vi "ArrDevMeasActionback.vi"(7 "DevId":i32, 8 "error in (no error)":errorcluster caption="entrée d'erreur (pas d'erreur)", 9 "CurvePointIndex":i32, 10 "AllPointIndex":i32, 11 "Device In":refnum<class "SymphonyCCD.lvclass"> caption="DNL_LabVIEW Object in") -> (0 "error out":errorcluster caption="sortie d'erreur", 1 "ArrDevDat":T1[](array[typedef]), 2 "MeasDatOut":dbl[][](array[numeric]), 3 "Device Out":refnum<class "SymphonyCCD.lvclass"> caption="DNL_LabVIEW Object out")   [LabVIEW 2019, in "SymphonyCCD.lvclass"]
uses:
  SymphonyCCD.lvclass
  C:/Programmes Labview/LabScanV1A/DevicesClass/BaseDevice/BaseDevice.lvclass
  Experiment Class/ArrDevData.ctl
  SymphonyCCD.lvclass/SymphonyCCD.ctl
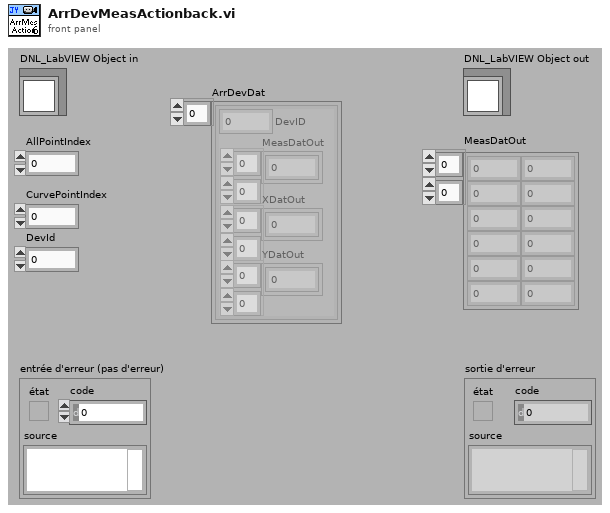
[diagram p1: front panel]
types:
  T1 = typedef "ArrDevData.ctl" = cluster{"MeasDatOut":dbl[][], "XDatOut":dbl[][], "YDatOut":dbl[][], "DevID":i32}
  T2 = cluster{"Message":string, "Data":variant, "Code":i32}
  T3 = typedef "SymphonyCCD.lvclass/SymphonyCCD_Func.ctl" = enum16{"AcqImageSim (Counts)", "AcqImage (Counts)"}
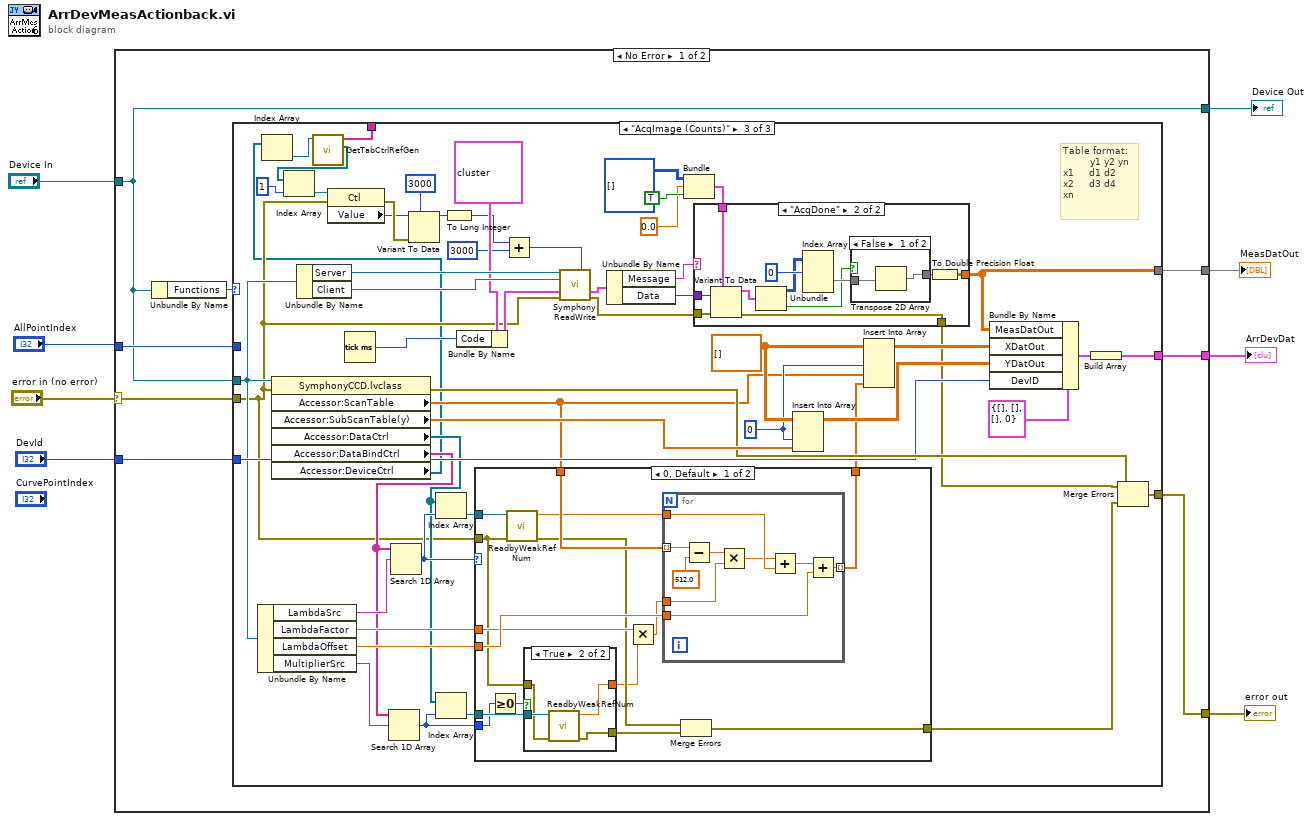
[diagram p0: block diagram]
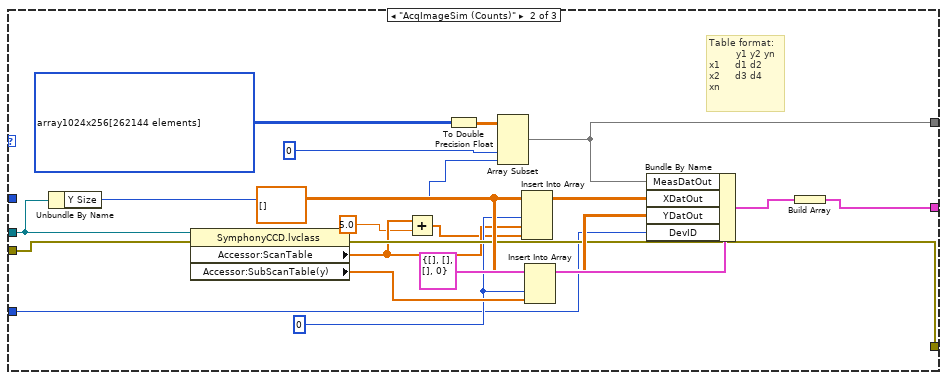
[diagram p3: hidden frame]
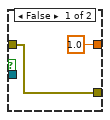
[diagram p4: hidden frame]
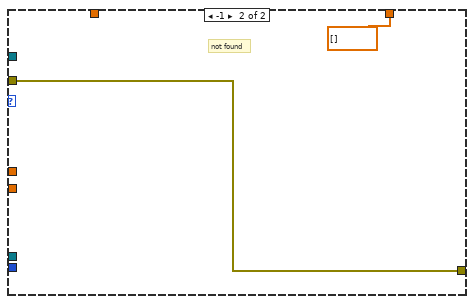
[diagram p5: hidden frame]
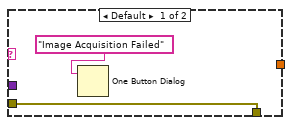
[diagram p6: hidden frame]
diagram:
  n1 = case shown="No Error" "error in (no error)" {
    selector: "error in (no error)" -> [w11 w141]
    tunnel: [w10 w141] -> w8
    tunnel: [w13 w140] -> w6
    tunnel: "Device In" -> [w13 w140]
    tunnel: [w14 _] -> w7
    tunnel: "AllPointIndex" -> [w15 _]
    tunnel: [w12 _] -> w2
    tunnel: "DevId" -> [w9 _]
    frame No Error {
      n2 = Unbundle By Name(w13) -> ("Functions"=w16:T3)
      n3 = case shown="\"AcqImage (Counts)\"" w16 {
        tunnel: w15 -> [_ _ _]
        tunnel: [_ w23 w72] -> w14
        tunnel: w13 -> [_ w26 w64]
        tunnel: [_ w30 w85] -> w12
        tunnel: w11 -> [w17 w29 w48]
        tunnel: [w17 w28 w71] -> w10
        tunnel: w9 -> [_ w21 w82]
        tunnel: [_ _ w39] -> _
        frame Default {
        }
        frame "AcqImageSim (Counts)" {
          w27 = 0 ("indice désactivé (col)")
          w31 = dbl[][] [] ("tableau")
          # "Table format: \n         y1 y2 yn\nx1     d1 d2\nx2     d3 d4\nxn"
          n4 = Unbundle By Name(w26) -> ("Y Size"=w22:i32)
          n5 = property class="SymphonyCCD.lvclass"(reference=w26, error in=w29) -> (error out=w28:errorcluster, "Accessor:ScanTable"=w20:dbl[], "Accessor:SubScanTable(y)"=w32:dbl[])  [unwired: 1 out]
          n6 = Add(x=w20, y=5.0) -> (x+y=w18:dbl[])
          n7 = To Double Precision Float(number=i32[][] array1024x256[262144 elements]) -> (double precision float=w25:dbl[][])
          n8 = Array Subset(array=w25, index (col)=0 ("indice"), length (col)=w22) -> (w23:dbl[][])  [unwired: 2 in]
          n9 = Insert Into Array(array=w31, index (col)=w27, new element #1=w20, new element #2=w18) -> (w34:dbl[][])  [unwired: 1 in]
          n10 = Insert Into Array(array=w31, index (col)=w27, new element=w32) -> (w33:dbl[][])  [unwired: 1 in]
          n11 = Bundle By Name(cluster=T1 {"MeasDatOut"=[], "XDatOut"=[], "YDatOut"=[], "DevID"=0} ("cluster de sortie"), "MeasDatOut"=w23, "XDatOut"=w34, "YDatOut"=w33, "DevID"=w21) -> (w35:T1)
          n12 = Build Array(w35) -> (w30:T1[])
        }
        frame "AcqImage (Counts)" {
          w83 = 0 ("indice désactivé (col)")
          w86 = dbl[][] [] ("tableau")
          # "Table format: \n         y1 y2 yn\nx1     d1 d2\nx2     d3 d4\nxn"
          n13 = Unbundle By Name(w64) -> ("LambdaSrc"=w61:string, "LambdaFactor"=w63:dbl, "LambdaOffset"=w62:dbl, "MultiplierSrc"=w56:string)
          n14 = property class="SymphonyCCD.lvclass"(reference=w64, error in=w48) -> (error out=w84:errorcluster, "Accessor:ScanTable"=w65:dbl[], "Accessor:SubScanTable(y)"=w87:dbl[], "Accessor:DataCtrl"=w57:refnum<vi>[], "Accessor:DataBindCtrl"=w55:string[], "Accessor:DeviceCtrl"=w42:refnum<vi>[])  [unwired: 1 out]
          n15 = Index Array(array=w42) -> (element=w41:refnum<vi>)  [unwired: 1 in]
          n16 = Unbundle By Name(w64) -> ("Server"=w81:refnum<k13>, "Client"=w80:refnum<k13>)
          n17 = call <userlib>:"GetTabCtrlRefGen.vi"("CommandRef"=w41) -> ("ControlsRefs"=w40:refnum<vi>[], "ControlsNames"=w39:string[])  [unwired: 8 in, 1 out]
          n18 = Index Array(array=w40, index=1) -> (element=w51:refnum<vi>)
          n19 = property class="Ctl"(reference=w51, error in=w48) -> (error out=w50:errorcluster, "Value"=w49:variant)  [unwired: 1 out]
          n20 = Tick Count (ms)() -> (millisecond timer value=w77:u32)
          n21 = Search 1D Array(1D array=w55, element=w56) -> (index of element=w54:i32)  [unwired: 1 in]
          n22 = Search 1D Array(1D array=w55, element=w61) -> (index of element=w58:i32)  [unwired: 1 in]
          n23 = Variant To Data(error in=w50, type=u32 3000 ("Read timeout ms(10000)"), Variant=w49) -> (data=w46:u32)  [unwired: 1 out]
          n24 = Index Array(array=w57, index=w58) -> (element=w60:refnum<vi>)
          n25 = Index Array(array=w57, index=w54) -> (element=w53:refnum<vi>)
          n26 = To Long Integer(number=w46) -> (32bit integer=w43:i32)
          n27 = Bundle By Name(cluster=T2 {"Message"="AcqImage", "Data"=variant, "Code"=0} ("Message In"), "Code"=w77) -> (w78:T2)
          n28 = case shown="0, Default" w58 {
            tunnel: w65 -> [w106 _]
            tunnel: w63 -> [w100 _]
            tunnel: w62 -> [w104 _]
            tunnel: w48 -> [w98 w122]
            tunnel: w60 -> [w105 _]
            tunnel: [w103 dbl[] []] -> w59
            tunnel: w54 -> [w92 _]
            tunnel: w53 -> [w101 _]
            tunnel: [w95 w122] -> w52
            frame 0, Default {
              n29 = Greater Or Equal To 0?(x=w92) -> (x >= 0?=w93:bool)
              n30 = call <userlib>:"ReadbyWeakRefNum.vi"("error in"=w98, "Control Ref"=w105) -> ("error out"=w97:errorcluster, "Valeur"=w102:dbl)  [unwired: 8 in]
              n31 = case shown="True" w93 {
                tunnel: w101 -> [_ w112]
                tunnel: w98 -> [w107 w111]
                tunnel: [w107 w110] -> w96
                tunnel: [1.0 ("Valeur") w109] -> w94
                frame False {
                }
                frame True {
                  n32 = call <userlib>:"ReadbyWeakRefNum.vi"("error in"=w111, "Control Ref"=w112) -> ("error out"=w110:errorcluster, "Valeur"=w109:dbl)  [unwired: 8 in]
                }
              }
              n33 = Multiply(x=w100, y=w94) -> (x*y=w99:dbl)
              n34 = for {
                tunnel: w106 -> [w117] mode=indexing
                tunnel: w102 -> [w121]
                tunnel: w99 -> [w119]
                tunnel: w104 -> [w114]
                tunnel: [w113] -> w103 mode=indexing
                n35 = Subtract(x=w117, y=512.0 ("x-1")) -> (x-y=w116:dbl)
                n36 = Multiply(x=w116, y=w119) -> (x*y=w120:dbl)
                n37 = Add(x=w120, y=w121) -> (x+y=w115:dbl)
                n38 = Add(x=w115, y=w114) -> (x+y=w113:dbl)
              }
              n39 = Merge Errors(w97, w96) -> (w95:errorcluster)
            }
            frame -1 {
              # "not found"
            }
          }
          n40 = Add(x=w43, y=3000 ("Read timeout ms(10000)")) -> (x+y=w44:i32)
          n41 = call <userlib>:"Symphony ReadWrite.vi"("ServerIn"=w81, "Read timeout ms(10000)"=w44, "ClientIn"=w80, "Message In"=w78, "ErrorIn (no error)"=w48) -> ("Data Out"=w76:T2, "error out"=w73:errorcluster)  [unwired: 7 in, 2 out]
          n42 = Unbundle By Name(w76) -> ("Message"=w75:string, "Data"=w74:variant)
          n43 = Bundle(i32[][][] [], 0.0, TRUE) -> (w68:cluster{i32[][][], dbl, bool})  [unwired: 1 in]
          n44 = case shown="\"AcqDone\"" w75 {
            tunnel: w74 -> [_ w136]
            tunnel: w68 -> [_ w134]
            tunnel: w73 -> [w124 w135]
            tunnel: [_ w132] -> w72
            tunnel: [w124 w131] -> w70
            frame Default {
              n45 = One Button Dialog(message="Image Acquisition Failed") -> ()  [unwired: 1 in, 1 out]
            }
            frame "AcqDone" {
              n46 = Variant To Data(error in=w135, type=w134, Variant=w136) -> (data=w130:cluster{i32[][][], dbl, bool}, error out=w131:errorcluster)
              n47 = Unbundle(w130) -> (w129:i32[][][], w126:bool)  [unwired: 1 out]
              n48 = Index Array(array=w129, index (dim 0)=0 ("indice (page)")) -> (element=w128:i32[][])  [unwired: 2 in]
              n49 = case shown="False" w126 {
                tunnel: w128 -> [w138 w139]
                tunnel: [w137 w139] -> w127
                frame False {
                  n50 = Transpose 2D Array(2D array=w138) -> (transposed array=w137:i32[][])
                }
                frame True {
                }
              }
              n51 = To Double Precision Float(number=w127) -> (double precision float=w132:dbl[][])
            }
          }
          n52 = Insert Into Array(array=w86, index (col)=w83, new element=w87) -> (w88:dbl[][])  [unwired: 1 in]
          n53 = Insert Into Array(array=w86, index (col)=w83, new element #1=w65, new element #2=w59) -> (w89:dbl[][])  [unwired: 1 in]
          n54 = Bundle By Name(cluster=T1 {"MeasDatOut"=[], "XDatOut"=[], "YDatOut"=[], "DevID"=0} ("cluster de sortie"), "MeasDatOut"=w72, "XDatOut"=w89, "YDatOut"=w88, "DevID"=w82) -> (w90:T1)
          n55 = Build Array(w90) -> (w85:T1[])
          n56 = Merge Errors(w70, w84, w52) -> (w71:errorcluster)
        }
      }
    }
    frame Error {
    }
  }
  "error out" <- w8
  "Device Out" <- w6
  "MeasDatOut" <- w7
  "ArrDevDat" <- w2
